vi "verify related subimage parameters.vi"(8 "error in (no error)":errorcluster, 11 "Simulated_CCD_Camera in":refnum<class "Sim_CCD.lvclass">) -> (0 "error out":errorcluster, 3 "Simulated_CCD_Camera out":refnum<class "Sim_CCD.lvclass">)   [LabVIEW 2018, in "Sim_CCD.lvclass"]
doc: "Verify the related parameters of the camera\n\nThere are some parameters of the camera operation mode that depend on the value provided for another parameter. This function verifies if these parameters are in agreement."
uses:
  Sim_CCD.lvclass
  Sim_CCD.lvclass/Sim_CCD.ctl
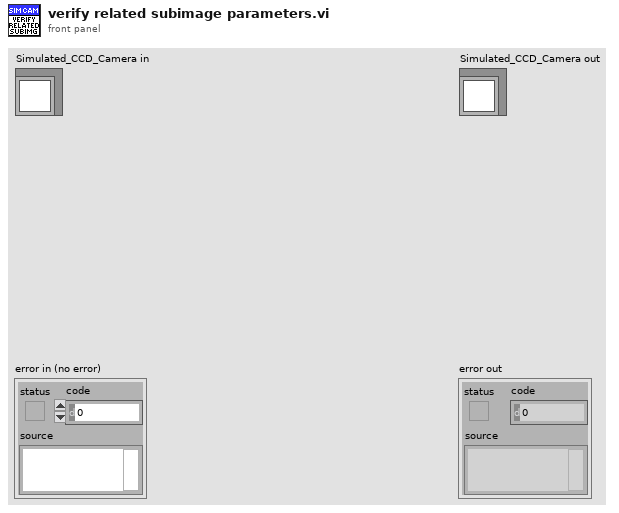
[diagram p1: front panel]
types:
  T1 = cluster{"PREAMP":u16, "READOUT_RATE":u16, "VERTICAL_SHIFT_SPEED":u16, "READ_MODE":u16, "VERTICAL_CLOCK_VOLTAGE":u16, "ACQUISITION_MODE":u16, "AD_CHANNEL":u16, "SHUTTER_TTL":u16, "SHUTTER_OPENING_TIME":u16, "SHUTTER_CLOSING_TIME":u16, "SHUTTER_MODE":u16, "TRIGGER_MODE":u16, "VBIN":u16, "INITIAL_LINE":u16, "INITIAL_COLUMN":u16, "FINAL_LINE":u16, "FINAL_COLUMN":u16, "HBIN":u16}
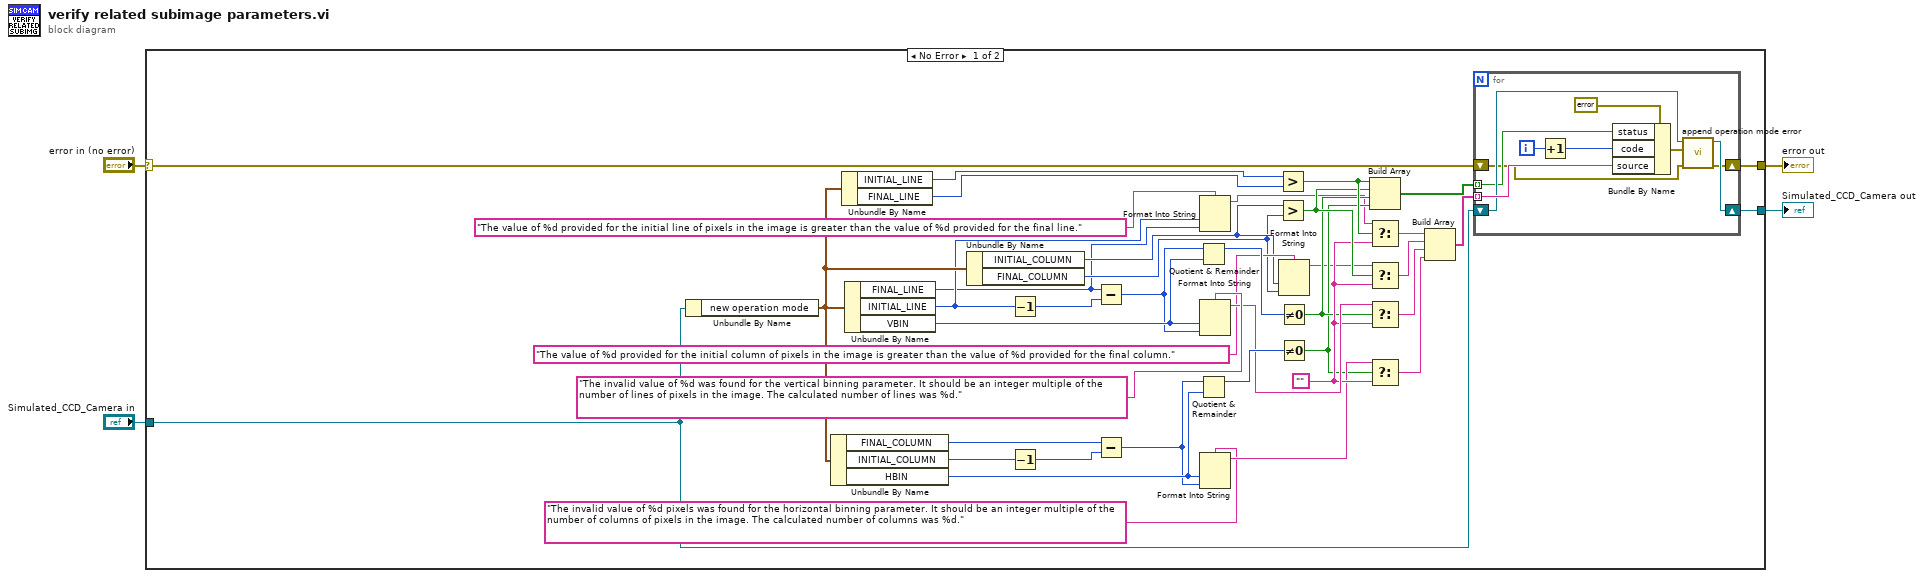
[diagram p0: block diagram]
diagram:
  n1 = case shown="No Error" "error in (no error)" {
    selector: "error in (no error)" -> [w27 w56]
    tunnel: [w26 w56] -> w3
    tunnel: [w28 w55] -> w1
    tunnel: "Simulated_CCD_Camera in" -> [w25 w55]
    frame No Error {
      w22 = ""
      n2 = Unbundle By Name(w25) -> ("new operation mode"=w30:T1)
      n3 = Unbundle By Name(w30) -> ("FINAL_COLUMN"=w34:u16, "INITIAL_COLUMN"=w33:u16, "HBIN"=w18:u16)
      n4 = Unbundle By Name(w30) -> ("INITIAL_LINE"=w44:u16, "FINAL_LINE"=w43:u16)
      n5 = Unbundle By Name(w30) -> ("FINAL_LINE"=w5:u16, "INITIAL_LINE"=w6:u16, "VBIN"=w19:u16)
      n6 = Unbundle By Name(w30) -> ("INITIAL_COLUMN"=w10:u16, "FINAL_COLUMN"=w9:u16)
      n7 = Decrement(x=w6) -> (x-1=w42:u16)
      n8 = Decrement(x=w33) -> (x-1=w35:u16)
      n9 = Subtract(x=w5, y=w42) -> (x-y=w15:u16)
      n10 = Subtract(x=w34, y=w35) -> (x-y=w14:u16)
      n11 = Quotient & Remainder(x=w15, y=w19) -> (x-y*floor(x/y)=w31:u16)  [unwired: 1 out]
      n12 = Quotient & Remainder(x=w14, y=w18) -> (x-y*floor(x/y)=w32:u16)  [unwired: 1 out]
      n13 = Format Into String(format string="The value of %d provided for the initial line of pixels in the image is greater than the value of %d provided for the final line.", w6, w5) -> (resulting string=w7:string)  [unwired: 2 in, 1 out]
      n14 = Format Into String(format string="The invalid value of %d was found for the vertical binning parameter. It should be an integer multiple of the number of lines of pixels in the image. The calculated number of lines was %d.", w19, w15) -> (resulting string=w23:string)  [unwired: 2 in, 1 out]
      n15 = Format Into String(format string="The invalid value of %d pixels was found for the horizontal binning parameter. It should be an integer multiple of the number of columns of pixels in the image. The calculated number of columns was %d.", w18, w14) -> (resulting string=w21:string)  [unwired: 2 in, 1 out]
      n16 = Greater?(x=w44, y=w43) -> (0:w38:bool)
      n17 = Greater?(x=w10, y=w9) -> (0:w37:bool)
      n18 = Format Into String(format string="The value of %d provided for the initial column of pixels in the image is greater than the value of %d provided for the final column.", w10, w9) -> (resulting string=w11:string)  [unwired: 2 in, 1 out]
      n19 = Not Equal To 0?(x=w31) -> (x != 0?=w17:bool)
      n20 = Not Equal To 0?(x=w32) -> (x != 0?=w16:bool)
      n21 = Build Array(w38, w37, w17, w16) -> (w29:bool[])
      n22 = Select(t=w7, s=w38, f=w22) -> (s? t:f=w41:string)
      n23 = Select(t=w11, s=w37, f=w22) -> (s? t:f=w40:string)
      n24 = Select(t=w23, s=w17, f=w22) -> (s? t:f=w39:string)
      n25 = Select(t=w21, s=w16, f=w22) -> (s? t:f=w13:string)
      n26 = Build Array(w41, w40, w39, w13) -> (w36:string[])
      n27 = for {
        tunnel: w36 -> [w54] mode=indexing
        tunnel: w29 -> [w50] mode=indexing
        shift-right: [w51] -> w28
        shift-left: w25 -> [w52]
        shift-right: [w48] -> w26
        shift-left: w27 -> [w49]
        i -> [w53]
        n28 = Increment(x=w53) -> (x+1=w47:i32)
        n29 = Bundle By Name(cluster=errorcluster {"status"=FALSE, "code"=0, "source"=""} ("error constant"), "status"=w50, "code"=w47, "source"=w54) -> (w45:errorcluster)
        n30 = call "append operation mode error.vi"("error in (no error)"=w49, "error"=w45, "Simulated_CCD_Camera in"=w52) -> ("error out"=w48:errorcluster, "Simulated_CCD_Camera out"=w51:refnum<class "Sim_CCD.lvclass">)  [unwired: 7 in]
      }
    }
    frame Error {
    }
  }
  "error out" <- w3
  "Simulated_CCD_Camera out" <- w1
